vi "Read Batch Profiles All.vi"(0 "Device ID (0)":i32, 1 "Timeout ms (5000)":u32=5000, 5 "Read Batch Profile Req":T3 {"Batch Pos" items=["CURRENT"=0, "SPECIFY"=2, "COMMITED"=3, "NEWEST PROFILE"=4]}, 7 "Read Profile Cnt":u32=1000, 11 "error in (no error)":errorcluster) -> (2 "Timeout ?":bool, 3 "Profile Info":T2, 4 "Device ID out":i32, 6 "Header Array":u32[][](array[numeric]), 8 "Height Profile Array":dbl[][](array[numeric]), 10 "Brightness Profile Array":u16[][](array[numeric]), 14 "Read Batch Profile Rsp":T1, 15 "error out":errorcluster)   [LabVIEW 2015, in "KEYENCE LJ-X8000A.lvlib"]
doc: "This function gets all batch profile data when bacth measurement is ON.\nThe height and brightness profile data are each stored in a simple array.\nThe height profile is in units of mm."
uses:
  KEYENCE LJ-X8000A.lvlib
  Clusters/Read Batch Profile Req for all read.ctl
  Constants/Batch Pos.ctl
  Clusters/Profile Info.ctl
  Clusters/Read Batch Profile Rsp.ctl
  Clusters/Read Batch Profile Req.ctl
panel:
  out "read profile counts(for debug)":u32[](array[numeric])
  out "read loop count(for debug)":i32
  out "”z—ñ":u32[](array[numeric])
  out "Process Time ms (for debug)":u32
  # "(c) 2019 KEYENCE CORPORATION.  ALL RIGHTS RESERVED."
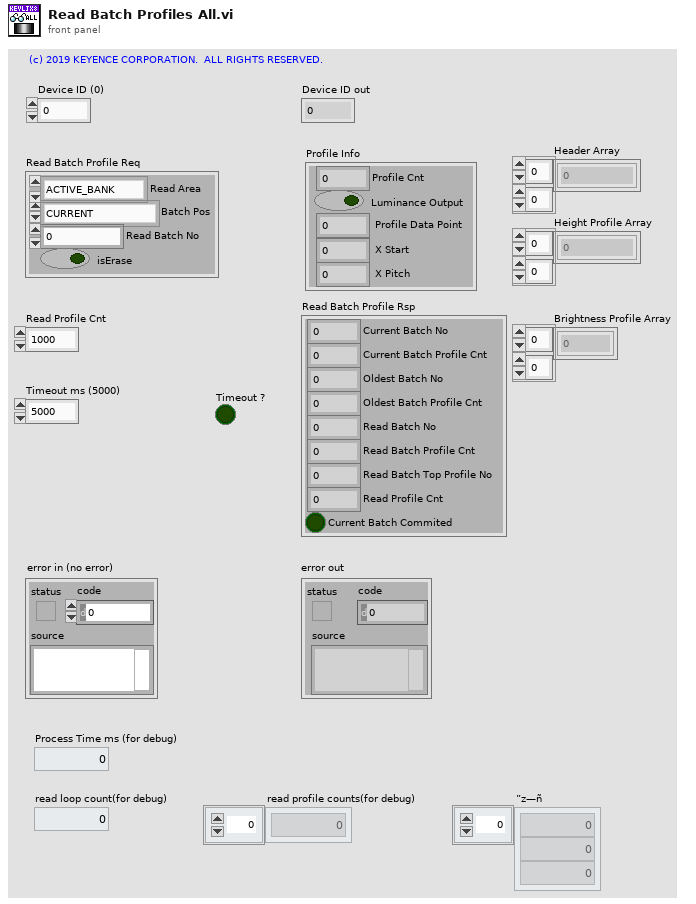
[diagram p1: front panel]
types:
  T1 = typedef "KEYENCE LJ-X8000A.lvlib/Read Batch Profile Rsp.ctl" = cluster{"Current Batch No":u32, "Current Batch Profile Cnt":u32, "Oldest Batch No":u32, "Oldest Batch Profile Cnt":u32, "Read Batch No":u32, "Read Batch Profile Cnt":u32, "Read Batch Top Profile No":u32, "Read Profile Cnt":u32, "Current Batch Commited":bool}
  T2 = typedef "KEYENCE LJ-X8000A.lvlib/Profile Info.ctl" = cluster{"Profile Cnt":u8, "Luminance Output":bool, " Profile Data Point":u16, " X Start":i32, " X Pitch":i32}
  T3 = typedef "KEYENCE LJ-X8000A.lvlib/Read Batch Profile Req for all read.ctl" = cluster{"Read Area":enum8{"ACTIVE_BANK", "INACTIVE_BANK"}, "Batch Pos":T4, "Read Batch No":u32, "isErase":bool}
  T4 = typedef "KEYENCE LJ-X8000A.lvlib/Batch Pos.ctl" = u8
  T5 = typedef "KEYENCE LJ-X8000A.lvlib/Read Batch Profile Req.ctl" = cluster{"Read Area":enum8{"ACTIVE_BANK", "INACTIVE_BANK"}, "Batch Pos":T4, "Read Batch No":u32, "Read Profile No.":u32, "Read Profile Cnt":u8, "isErase":bool}
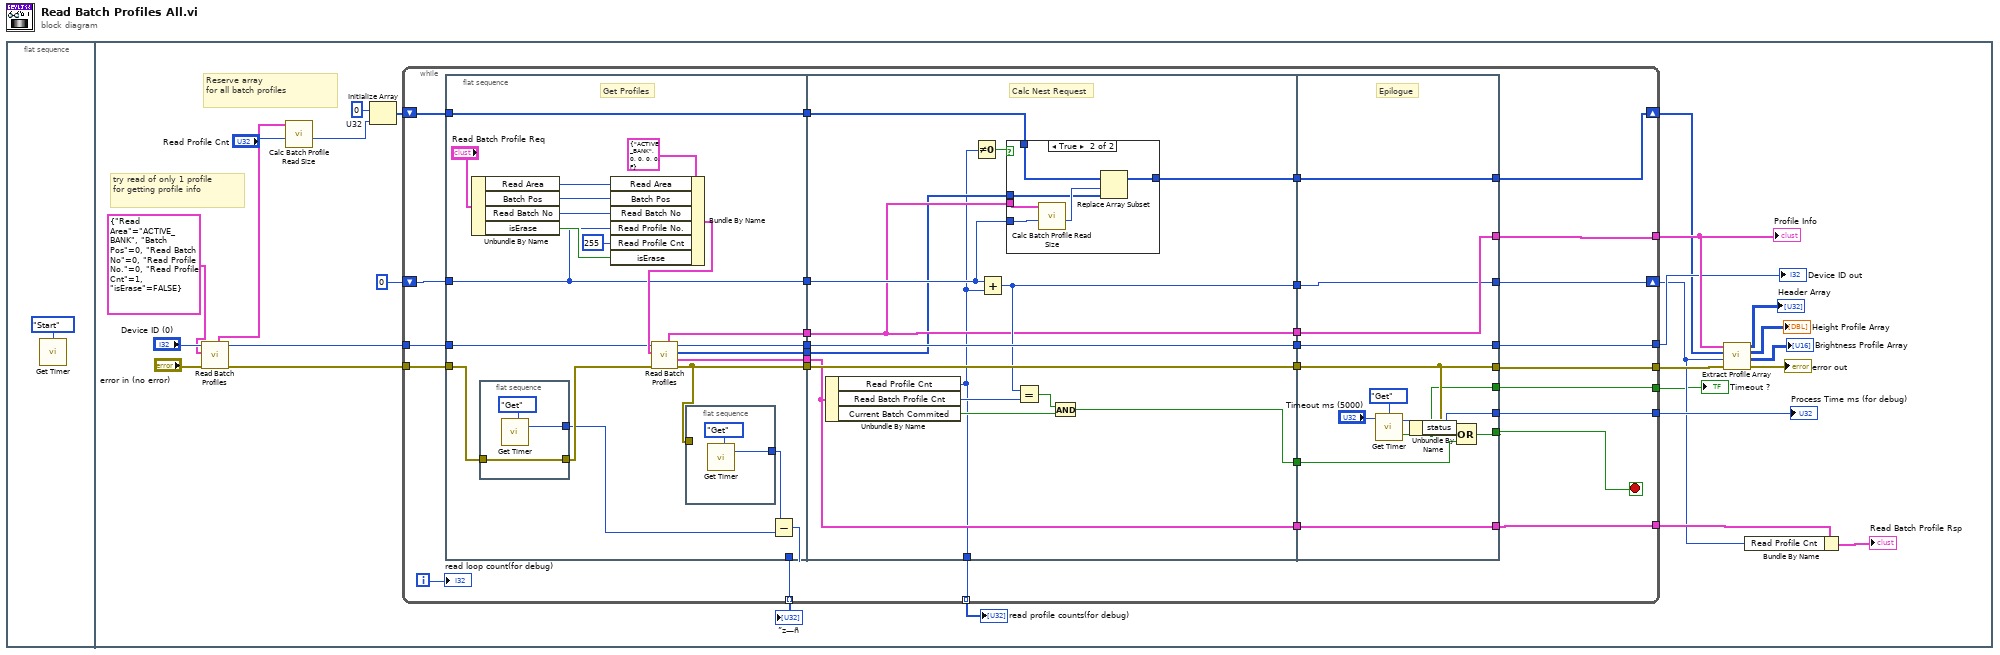
[diagram p0: block diagram]
diagram:
  n1 = flat-sequence {
    frame #0 {
      n2 = call "Get Timer.vi"("Mode"=enum8{"Start", "Get"}."Start") -> ()  [unwired: 3 in, 2 out]
    }
    frame #1 {
      w20 = u32 0  # U32
      # "Reserve array\nfor all batch profiles"
      # "try read of only 1 profile \nfor getting profile info"
      n3 = call "Read Batch Profiles.vi"("error in (no error)"="error in (no error)", "Read Batch Profile Req"=T5 {"Read Area"=enum."ACTIVE_BANK", "Batch Pos"=0, "Read Batch No"=0, "Read Profile No."=0, "Read Profile Cnt"=1, "isErase"=FALSE}, "Device ID (0)"="Device ID (0)") -> ("error out"=w19:errorcluster, "Device ID out"=w18:i32, "Profile Info"=w22:T2)  [unwired: 4 in, 2 out]
      n4 = call "Calc Batch Profile Read Size.vi"("Read Profile Cnt"="Read Profile Cnt", "Profile Info"=w22) -> ("Required Size(DWORD)"=w16:u32)  [unwired: 8 in, 1 out]
      n5 = Initialize Array(w20, w16) -> (w17:u32[])
      n6 = while {
        shift-right: [w42] -> w5
        shift-left: u32 0 ("Read Profile No.") -> [w55]
        tunnel: [w56] -> w26
        tunnel: [w54] -> w15
        tunnel: [w53] -> w13
        tunnel: [w52] -> w6
        tunnel: w19 -> [w39]
        tunnel: w18 -> [w40]
        shift-right: [w34] -> w12
        shift-left: w17 -> [w38]
        tunnel: [w32] -> w8
        tunnel: [w31] -> w4 mode=indexing
        tunnel: [w29] -> w3 mode=indexing
        tunnel: [w28] -> w2
        i -> [w30]
        stop <- w57 stop-if-true
        n7 = flat-sequence {
          tunnel: [w63] -> w51
          tunnel: w55 -> [w69]
          tunnel: [w72] -> w49
          tunnel: [w71] -> w47
          tunnel: [w70] -> w45
          tunnel: [w69] -> w44
          tunnel: w40 -> [w67]
          tunnel: w39 -> [w62]
          tunnel: w38 -> [w66]
          tunnel: [w66] -> w37
          tunnel: [w65] -> w36
          tunnel: [w58] -> w31
          tunnel: w51 -> [w98]
          tunnel: [w98] -> w50
          tunnel: w49 -> [w89]
          tunnel: [w89] -> w48
          tunnel: w47 -> [w97]
          tunnel: [w97] -> w46
          tunnel: w45 -> [w85]
          tunnel: w44 -> [w90]
          tunnel: [w96] -> w43
          tunnel: [w92] -> w41
          tunnel: w37 -> [w88]
          tunnel: w36 -> [w87]
          tunnel: [w86] -> w35
          tunnel: [w85] -> w33
          tunnel: [w84] -> w29
          tunnel: w50 -> [w114]
          tunnel: [w118] -> w57
          tunnel: [w117] -> w56
          tunnel: w48 -> [w116]
          tunnel: [w116] -> w54
          tunnel: [w115] -> w53
          tunnel: w46 -> [w115]
          tunnel: [w114] -> w52
          tunnel: w43 -> [w113]
          tunnel: [w113] -> w42
          tunnel: w41 -> [w112]
          tunnel: w35 -> [w111]
          tunnel: [w111] -> w34
          tunnel: w33 -> [w110]
          tunnel: [w110] -> w32
          tunnel: [w107] -> w28
          frame #0 {
            # "Get Profiles"
            n8 = Unbundle By Name("Read Batch Profile Req") -> ("Read Area"=w74:enum8{"ACTIVE_BANK", "INACTIVE_BANK"}, "Batch Pos"=w68:T4, "Read Batch No"=w75:u32, "isErase"=w76:bool)
            n9 = flat-sequence {
              tunnel: [w80] -> w59
              tunnel: w62 -> [w79]
              tunnel: [w79] -> w61
              frame #0 {
                n10 = call "Get Timer.vi"("Mode"=enum8{"Start", "Get"}."Get") -> ("Time(ms)"=w80:u32)  [unwired: 3 in, 1 out]
              }
            }
            n11 = Bundle By Name(cluster=T5 {"Read Area"=enum."ACTIVE_BANK", "Batch Pos"=0, "Read Batch No"=0, "Read Profile No."=0, "Read Profile Cnt"=0, "isErase"=FALSE} ("Read Batch Profile Req"), "Read Area"=w74, "Batch Pos"=w68, "Read Batch No"=w75, "Read Profile No."=w69, "Read Profile Cnt"=u8 255, "isErase"=w76) -> (w73:T5)
            n12 = call "Read Batch Profiles.vi"("error in (no error)"=w61, "Read Batch Profile Req"=w73, "Device ID (0)"=w67) -> ("error out"=w63:errorcluster, "Read Batch Profile Rsp"=w70:T1, "Profile Data"=w65:u32[], "Device ID out"=w71:i32, "Profile Info"=w72:T2)  [unwired: 4 in]
            n13 = flat-sequence {
              tunnel: w63 -> [_]
              tunnel: [w82] -> w60
              frame #0 {
                n14 = call "Get Timer.vi"("Mode"=enum8{"Start", "Get"}."Get") -> ("Time(ms)"=w82:u32)  [unwired: 3 in, 1 out]
              }
            }
            n15 = Subtract(x=w60, y=w59) -> (x-y=w58:u32)
          }
          frame #1 {
            # "Calc Nest Request"
            n16 = Unbundle By Name(w85) -> ("Read Profile Cnt"=w84:u32, "Read Batch Profile Cnt"=w95:u32, "Current Batch Commited"=w94:bool)
            n17 = Not Equal To 0?(x=w84) -> (x != 0?=w91:bool)
            n18 = Add(x=w90, y=w84) -> (x+y=w96:u32)
            n19 = case shown="True" w91 {
              tunnel: w90 -> [_ w105]
              tunnel: w89 -> [_ w104]
              tunnel: w88 -> [w99 w103]
              tunnel: w87 -> [_ w101]
              tunnel: [w99 w100] -> w86
              frame False {
              }
              frame True {
                n20 = call "Calc Batch Profile Read Size.vi"("Read Profile Cnt"=w105, "Profile Info"=w104) -> ("Required Size(DWORD)"=w102:u32)  [unwired: 8 in, 1 out]
                n21 = Replace Array Subset(array=w103, new element=w101, index=w102) -> (w100:u32[])
              }
            }
            n22 = Equal?(x=w96, y=w95) -> (x = y?=w93:bool)
            n23 = And(x=w93, y=w94) -> (x .and. y?=w92:bool)
          }
          frame #2 {
            # "Epilogue"
            n24 = call "Get Timer.vi"("Mode"=enum8{"Start", "Get"}."Get", "Timeout(ms)"="Timeout ms (5000)") -> ("Timeout ?"=w107:bool, "Time(ms)"=w117:u32)  [unwired: 2 in]
            n25 = Unbundle By Name(w114) -> ("status"=w106:bool)
            n26 = Compound Arithmetic op=OR ("¡Z")(w106, w107, w112) -> (w118:bool)
          }
        }
        "read loop count(for debug)" <- w30
      }
      "Process Time ms (for debug)" <- w26
      "Profile Info" <- w15
      "Device ID out" <- w13
      "”z—ñ" <- w4
      "read profile counts(for debug)" <- w3
      "Timeout ?" <- w2
      n27 = call "Extract Profile Array.vi"("error in (no error)"=w6, "Profile Cnt"=w5, "Profile Data"=w12, "Profile Info"=w15) -> ("error out"=→"error out":errorcluster, "Luminance Profile Array"=→"Brightness Profile Array":u16[][], "16位forImage"=→"Height Profile Array":i16[][], "Header Array"=→"Header Array":u32[][])  [unwired: 4 in]
      n28 = Bundle By Name(cluster=w8, "Read Profile Cnt"=w5) -> (→"Read Batch Profile Rsp":T1)
    }
  }
